vi "Configure Laser Sensitivity.vi"(8 "error in (no error)":errorcluster, 10 "Sensitivity Mode (0: Normal mode)":u32(ring) items=["Normal mode", "High sensitivity mode"], 11 "VISA resource name":refnum<visa-resource-name>) -> (0 "error out":errorcluster, 3 "VISA resource name out":refnum<visa-resource-name>)   [LabVIEW 2011, in "Hokuyo URG Series.lvlib"]
doc: "This command will switch between high sensitivity and normal sensitivity modes. If the laser is already running in the selected sensitivity mode, an error will be returned.\n\nThis may not be supported on all models and has not been tested by National Instruments. Refer to product manual for information on this mode."
uses:
  Hokuyo URG Series.lvlib
panel:
  # "This function has not been tested \nby National Instruments"
  # "Sensor’s detection ability will increase about 20% in the high sensitivity mode. However there may be chances of measurement errors due to strong reflective objects near 22m. \n\nNote: This command is not compatible in all versions of UTM-30LX and URG-04LX with firmware versions earlier than 3.2.00."
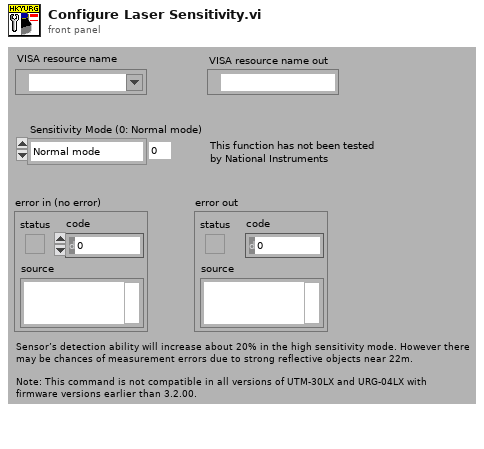
[diagram p1: front panel]
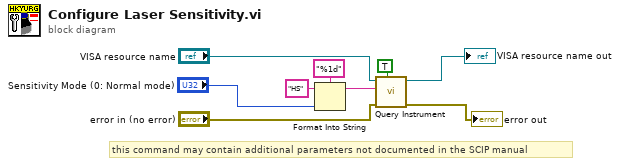
[diagram p0: block diagram]
diagram:
  # "this command may contain additional parameters not documented in the SCIP manual"
  n1 = Format Into String(format string="%1d", initial string="HS" ("command"), "Sensitivity Mode (0: Normal mode)") -> (resulting string=w5:string)  [unwired: 1 in, 1 out]
  n2 = call "Query Instrument.vi"("Error Query (Enabled)"=TRUE, "error in"="error in (no error)", "Command"=w5, "VISA Resource Name"="VISA resource name") -> ("error out"=→"error out":errorcluster, "VISA Resource Name Out"=→"VISA resource name out":refnum<visa-resource-name>)  [unwired: 5 in, 1 out]
